vi "Gran method.vi"(0 "Serial Port":refnum<visa-resource-name>, 1 "seconds/data point":u16=10 min=1 max=9999 step=1, 2 "ok":bool, 3 "auto/manual":bool, 4 "Channel A":enum16{"OFF", "pH", "mV", "ion", "conductivity"}(ring)=enum."pH", 5 "Channel B":enum16{"OFF", "pH", "mV", "ion"}(ring)) -> (14 "canceled":bool=TRUE, 15 "seconds/data point out":u16=10 min=1 max=9999 step=1, 16 "2nd channel":bool=TRUE, 17 "auto/manual out":bool=TRUE, 18 "Channel A out":enum16{"OFF", "pH", "mV", "ion", "conductivity"}(ring)=enum."pH", 19 "Channel B out":enum16{"OFF", "pH", "mV", "ion"}(ring)=enum."pH")   [LabVIEW 2010]
panel:
  out "setting up meter":string="Sending method to meter. Please wait. Do not change the display of the meter after setting the method!"
  in  "probe type":string[](array[string])=["", "A", "B", "C", "D"]
  in  "cancel":bool
  out "channels":T1(ring)
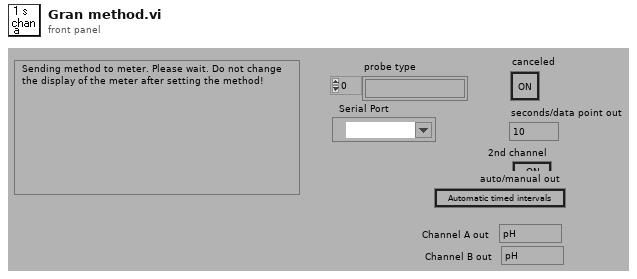
[diagram p1: front panel]
types:
  T1 = enum16{"channel A", "Channel B", "Channel A and B"}
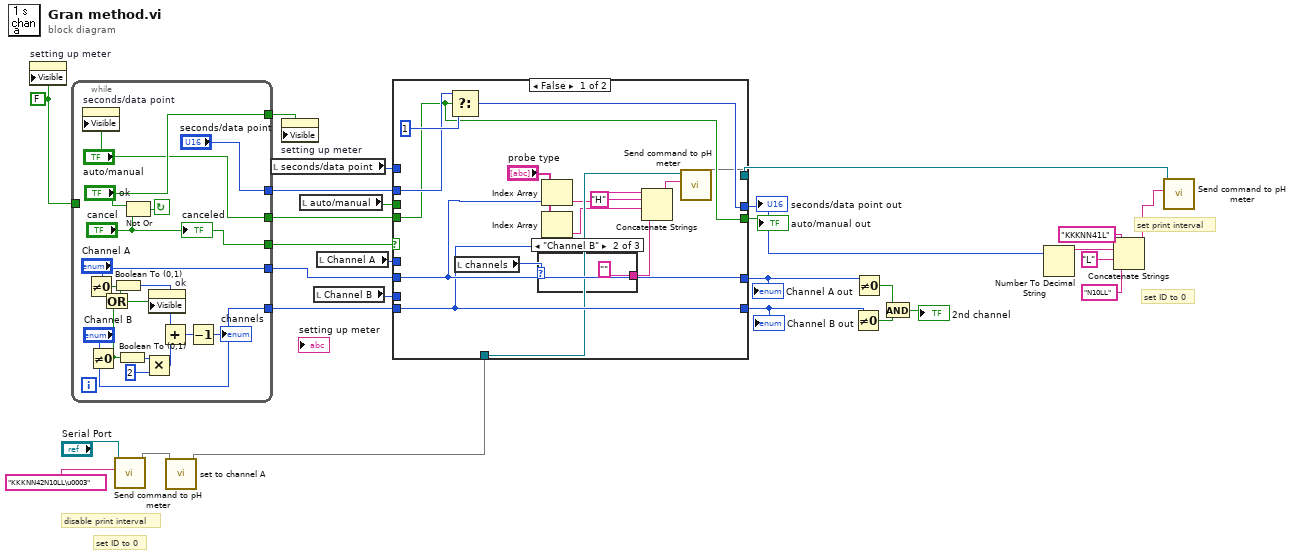
[diagram p0: block diagram]
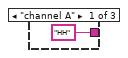
[diagram p2: hidden frame]
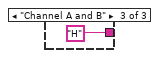
[diagram p3: hidden frame]
diagram:
  w13 = FALSE
  # "set print interval"
  # "set ID to 0"
  # "set ID to 0"
  # "disable print interval"
  n1 = property on="setting up meter" class="Str"("Visible"=w13) -> ()  [unwired: 2 in, 2 out]
  n2 = while {
    tunnel: ["ok"] -> w9
    tunnel: w13 -> [_]
    tunnel: ["Channel B"] -> w19
    tunnel: ["Channel A"] -> w20
    tunnel: ["auto/manual"] -> w23
    tunnel: ["seconds/data point"] -> w27
    tunnel: ["cancel"] -> w28
    stop <- w29 continue-if-true
    n3 = property on="seconds/data point" class="DigNum (strict)"("Visible"="auto/manual") -> ()  [unwired: 2 in, 2 out]
    n4 = Not Equal To 0?(x="Channel A") -> (x != 0?=w32:bool)
    n5 = Not Equal To 0?(x="Channel B") -> (x != 0?=w31:bool)
    n6 = Or(x=w32, y=w31) -> (x .or. y?=w33:bool)
    n7 = Boolean To (0,1)(Boolean=w32) -> (0, 1=w34:i16)
    n8 = Boolean To (0,1)(Boolean=w31) -> (0, 1=w37:i16)
    n9 = Not Or(1:"cancel", 2:"ok") -> (0:w29:bool)
    n10 = Multiply(x=w37, y=2) -> (x*y=w36:i32)
    n11 = property on="ok" class="Bool"("Visible"=w33) -> ()  [unwired: 2 in, 2 out]
    n12 = Add(x=w34, y=w36) -> (x+y=w41:i32)
    n13 = Decrement(x=w41) -> (x-1=→"channels":i32)
    "canceled" <- "cancel"
  }
  n14 = call "Send command to pH meter"("string to write"="KKKNN42N10LL\u0003", 11:"Serial Port") -> (3:w11)  [unwired: 7 in, 2 out]
  n15 = call "set to channel A.vi"(11:w11) -> (3:w8)  [unwired: 9 in, 1 out]
  n16 = local read "seconds/data point"() -> (w24:u16)
  n17 = property on="setting up meter" class="Str"("Visible"=w9) -> ()  [unwired: 2 in, 2 out]
  n18 = local read "auto/manual"() -> (w21:bool)
  n19 = local read "Channel B"() -> (w17:enum16{"OFF", "pH", "mV", "ion"})
  n20 = local read "Channel A"() -> (w18:enum16{"OFF", "pH", "mV", "ion", "conductivity"})
  n21 = case shown="False" w28 {
    tunnel: [w46 w67] -> w1
    tunnel: w27 -> [w48 _]
    tunnel: w24 -> [_ w67]
    tunnel: w23 -> [w47 _]
    tunnel: [w47 w66] -> w22
    tunnel: w21 -> [_ w66]
    tunnel: w20 -> [w59 _]
    tunnel: w19 -> [w58 _]
    tunnel: [w59 w65] -> w14
    tunnel: w18 -> [_ w65]
    tunnel: [w58 w64] -> w15
    tunnel: w17 -> [_ w64]
    tunnel: w8 -> [w57 w63]
    tunnel: [w45 w63] -> w2
    frame False {
      n22 = Select(t=w48, s=w47, f=u16 1) -> (s? t:f=w46:u16)
      n23 = local read "channels"() -> (w54:T1)
      n24 = case shown="\"Channel B\"" w54 {
        tunnel: ["HH" "" "H"] -> w53
        frame "channel A" {
        }
        frame "Channel B" {
        }
        frame "Channel A and B" {
        }
      }
      n25 = Index Array(array="probe type", index=w59) -> (element=w49:string)
      n26 = Index Array(array="probe type", index=w58) -> (element=w51:string)
      n27 = Concatenate Strings(w49, "H", w51, w53) -> (w55:string)
      n28 = call "Send command to pH meter"("string to write"=w55, 11:w57) -> (3:w45)  [unwired: 7 in, 2 out]
    }
    frame True {
    }
  }
  "seconds/data point out" <- w1
  "Channel A out" <- w14
  "Channel B out" <- w15
  "auto/manual out" <- w22
  n29 = Not Equal To 0?(x=w15) -> (x != 0?=w26:bool)
  n30 = Not Equal To 0?(x=w14) -> (x != 0?=w25:bool)
  n31 = And(x=w25, y=w26) -> (x .and. y?=→"2nd channel":bool)
  n32 = Number To Decimal String(number=w1) -> (decimal integer string=w5:string)  [unwired: 1 in]
  n33 = Concatenate Strings("KKKNN41L", w5, "L", "N10LL") -> (w7:string)
  n34 = call "Send command to pH meter"("string to write"=w7, 11:w2) -> ()  [unwired: 8 in, 2 out]
